vi "myRIO v1.0 Generate Register Values PWM.vi"(8 "error in (no error)":errorcluster, 11 "Frequency (Hz)":dbl) -> (0 "error out":errorcluster, 1 "PWM.CS":u8 format="%.0b", 2 "PWM.CNFG":u8, 3 "PWM.MAX":u16, 5 "Actual Frequency (Hz)":dbl)   [LabVIEW 2021]
uses:
  <vilib>/myRIO/Common/Instrument Driver Framework/Utilities/typedefs/Clock Calculation Parameters.ctl
  <vilib>/myRIO/Common/Instrument Driver Framework/Utilities/vis/Calculate TOP (Phase Correct Mode).vi
  <vilib>/myRIO/Common/Instrument Driver Framework/Utilities/vis/Calculate TOP (Normal Mode).vi
  <vilib>/myRIO/Common/Instrument Driver Framework/Utilities/vis/Calculate Frequency (Phase Correct Mode).vi
  <vilib>/myRIO/Common/Instrument Driver Framework/Utilities/vis/Calculate Frequency (Normal Mode).vi
  <vilib>/Utility/error.llb/Error Cluster From Error Code.vi
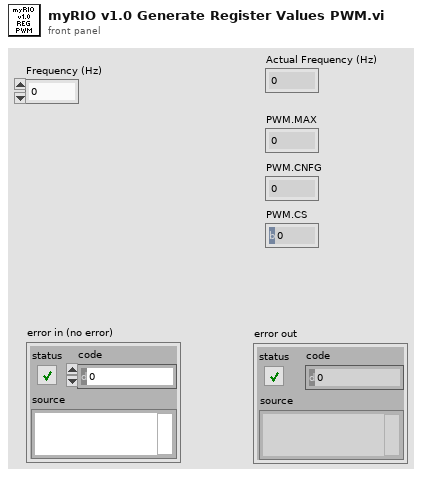
[diagram p1: front panel]
types:
  T1 = typedef "Clock Calculation Parameters.ctl" = cluster{"Base Clock Frequency (Hz)":dbl, "Max Counter Value":u32, "Min Counter Value":u32}
  T2 = typedef "Clock Settings.ctl" = cluster{"Clock Divisor":u32, "TOP":u32, "Actual Frequency (Hz)":dbl}
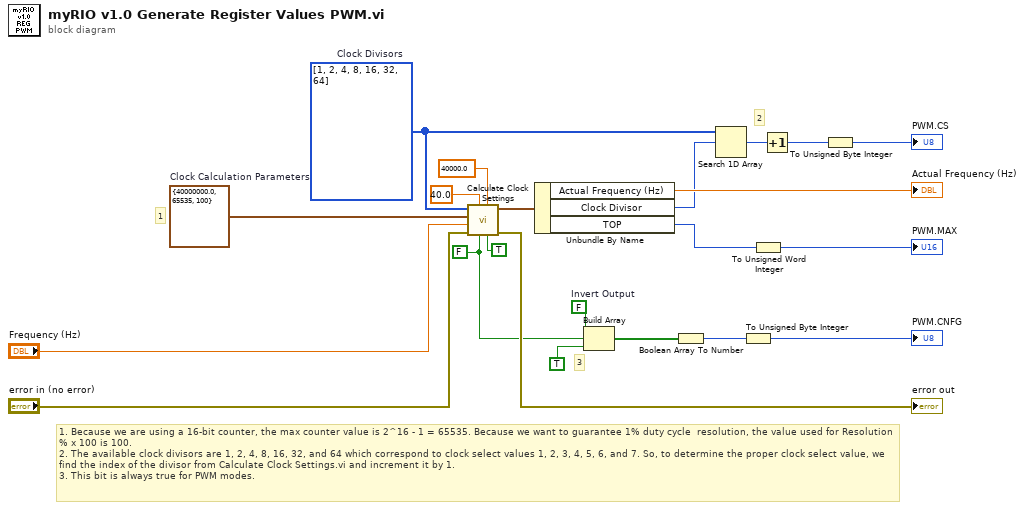
[diagram p0: block diagram]
diagram:
  w7 = FALSE  # Invert Output
  w8 = FALSE ("Phase Correct Mode?")
  w10 = T1 {"Base Clock Frequency (Hz)"=40000000.0, "Max Counter Value"=65535, "Min Counter Value"=100}  # Clock Calculation Parameters
  w9 = u32[] [1, 2, 4, 8, 16, 32, 64]  # Clock Divisors
  # "3"
  # "2"
  # "1"
  # "1. Because we are using a 16-bit counter, the max counter value is 2^16 - 1 = 65535. Because we want to guarantee 1% duty cycle  resolution, the value used for Resolution % x 100 is 100.\n2. The available clock divisors are 1, 2, 4, 8, 16, 32, and 64 which correspond to clock select values 1, 2, 3, 4, 5, 6, and 7. So, to determine the proper clock select value, we find the index of the divisor from Calculate Clock Settings.vi and increment it by 1.\n3. This bit is always true for PWM modes."
  n1 = call <vilib>:"Calculate Clock Settings.vi"("Coerce Range?"=TRUE, "Max Frequency (Hz)"=40000.0 ("upper limit"), "Phase Correct Mode?"=w8, "Min Frequency (Hz)"=40.0 ("lower limit"), "error in (no error)"="error in (no error)", "Requested Frequency (Hz)"="Frequency (Hz)", "Clock Calculation Parameters"=w10, "Clock Divisors"=w9) -> ("error out"=→"error out":errorcluster, "Frequency Configuration"=w19:T2)  [unwired: 2 in]
  n2 = Unbundle By Name(w19) -> ("Actual Frequency (Hz)"=→"Actual Frequency (Hz)":dbl, "Clock Divisor"=w16:u32, "TOP"=w17:u32)
  n3 = Build Array(w7, w8, TRUE ("element")) -> (w13:bool[])
  n4 = Boolean Array To Number(Boolean array=w13) -> (number=w15:u32)
  n5 = Search 1D Array(1D array=w9, element=w16) -> (index of element=w18:i32)  [unwired: 1 in]
  n6 = To Unsigned Byte Integer(number=w15) -> (unsigned 8bit integer=→"PWM.CNFG":u8)
  n7 = To Unsigned Word Integer(number=w17) -> (unsigned 16bit integer=→"PWM.MAX":u16)
  n8 = Increment(x=w18) -> (x+1=w3:i32)
  n9 = To Unsigned Byte Integer(number=w3) -> (unsigned 8bit integer=→"PWM.CS":u8)
